vi "refresh table model.vi"(7 "engine configuration":refnum<class "engine configuration.lvclass">, 8 "error in":errorcluster, 9 "avail tags":refnum<vi>, 10 "chan table":refnum<vi>, 11 "bin datalogger configuration":refnum<class "Binary datalogger configuration.lvclass">) -> (0 "error out":errorcluster, 3 "bin datalogger configuration out":refnum<class "Binary datalogger configuration.lvclass">, 5 "engine configuration out":refnum<class "engine configuration.lvclass">)   [LabVIEW 2013, in "Binary datalogger editor node.lvclass"]
uses:
  Binary datalogger editor node.lvclass
  module/configuration/Binary datalogger configuration.lvclass
  <vilib>/NI/Module Execution Interface/Engine Configuration/engine configuration.lvclass
  <vilib>/NI/Configuration Framework/serializable configuration/NISE_CEF_serializable configuration.lvclass/NISE_CEF_serializable configuration.ctl
  module/configuration/Binary datalogger configuration.lvclass/Binary datalogger configuration.ctl
  <vilib>/NI/Tag Bus/tag/tag descriptor.lvclass/tag descriptor.ctl
  <vilib>/NI/Module Execution Interface/Engine Configuration/engine configuration.lvclass/engine configuration.ctl
  <vilib>/NI/Tag Bus/tag/write tag name.vi
  <vilib>/NI/Tag Bus/tag/read tag name.vi
  <vilib>/NI/Tag Bus/tag/read data type.vi
  <vilib>/NI/Configuration Framework/serializable configuration/Read UID.vi
  module/configuration/Read channels.vi
  <vilib>/Utility/LVClass/Get LV Class Name.vi
  <vilib>/NI/Configuration Framework/error generator/NISE_error generator.vi
  <vilib>/NI/Tag Bus Module Framework/channel/TBM channel.lvclass
  <vilib>/NI/Tag Bus/tag/tag descriptor.lvclass
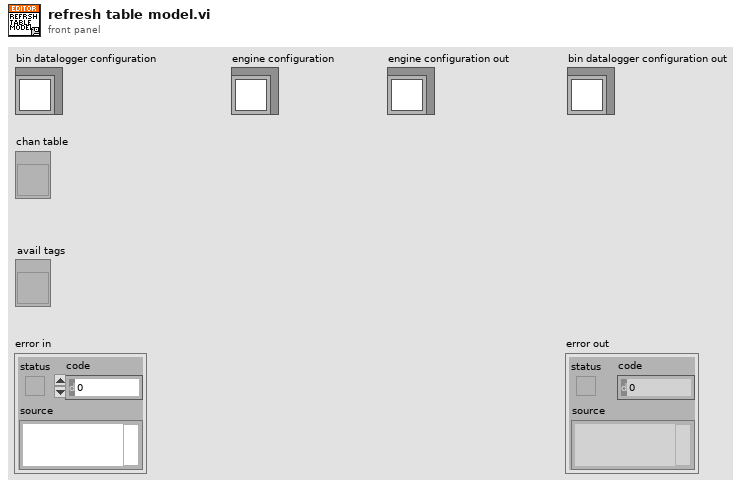
[diagram p1: front panel]
types:
  T1 = typedef "tag bus.lvlib/tag descriptor.lvclass/Data Type.ctl" = enum16{"Double", "Single", "I64", "I32", "I16", "I8", "U64", "U32", "U16", "U8", "Boolean", "String", "Array of Double", "Array of Single", "Array of I64", "Array of I32", "Array of I16", "Array of I8", "Array of U64", "Array of U32", "Array of U16", "Array of U8", "Array of Boolean", "Array of String"}
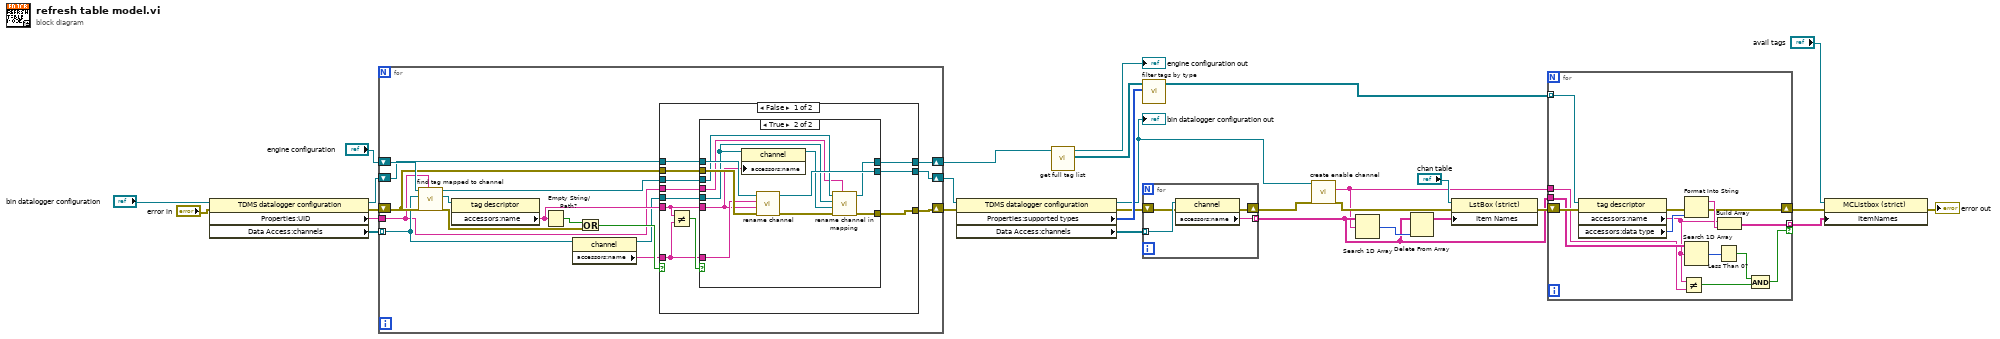
[diagram p0: block diagram]
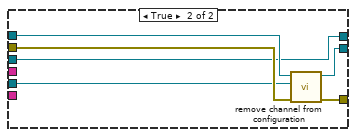
[diagram p3: hidden frame]
diagram:
  n1 = property class="TDMS datalogger configuration"(reference="bin datalogger configuration", error in="error in") -> (reference out=w24:refnum<class "Binary datalogger configuration.lvclass">, error out=w26:errorcluster, "Properties:UID"=w20:string, "Data Access:channels"=w27:refnum<class "TBM channel.lvclass">[])
  n2 = for {
    tunnel: w27 -> [w37] mode=indexing
    shift-right: [w32] -> w8
    shift-left: "engine configuration" -> [w45]
    shift-right: [w42] -> w23
    shift-left: w24 -> [w40]
    tunnel: w20 -> [w31]
    shift-right: [w41] -> w22
    shift-left: w26 -> [w38]
    n3 = call <vilib>:"find tag mapped to channel.vi"("owner"=w31, "error in"=w38, "channel"=w37, "engine configuration in"=w45) -> ("error out"=w36:errorcluster, "tag"=w44:refnum<class "tag descriptor.lvclass">, "engine configuration out"=w33:refnum<class "engine configuration.lvclass">)  [unwired: 5 in]
    n4 = property class="tag descriptor"(reference=w44) -> ("accessors:name"=w34:string)  [unwired: 1 in, 2 out]
    n5 = Empty String/Path?(string/path=w34) -> (empty?=w43:bool)
    n6 = property class="channel"(reference=w37) -> (reference out=w30:refnum<class "TBM channel.lvclass">, "accessors:name"=w35:string)  [unwired: 1 in, 1 out]
    n7 = Or(x=w43, y=w36) -> (x .or. y?=w39:bool)
    n8 = case shown="False" w39 {
      tunnel: [w53 w77] -> w42
      tunnel: [w56 w76] -> w41
      tunnel: w38 -> [w55 w75]
      tunnel: w40 -> [w54 w74]
      tunnel: w30 -> [w46 w73]
      tunnel: w35 -> [w51 _]
      tunnel: w34 -> [w50 _]
      tunnel: w33 -> [w49 w72]
      tunnel: [w48 w72] -> w32
      tunnel: w31 -> [w47 _]
      frame False {
        n9 = Not Equal?(x=w50, y=w51) -> (x != y?=w52:bool)
        n10 = case shown="True" w52 {
          tunnel: [w59 w64] -> w56
          tunnel: w55 -> [w59 w70]
          tunnel: w54 -> [w58 w71]
          tunnel: [w58 w69] -> w53
          tunnel: w51 -> [_ w68]
          tunnel: w50 -> [_ w61]
          tunnel: w49 -> [w57 w67]
          tunnel: [w57 w66] -> w48
          tunnel: w47 -> [_ w63]
          tunnel: w46 -> [_ w62]
          frame False {
          }
          frame True {
            n11 = property class="channel"(reference=w62, "accessors:name"=w61) -> (reference out=w60:refnum<class "TBM channel.lvclass">)  [unwired: 1 in, 1 out]
            n12 = call "rename channel.vi"("error in"=w70, "new name"=w61, "old name"=w68, "bin datalogger configuration in"=w71) -> ("error out"=w65:errorcluster, "bin datalogger configuration out"=w69:refnum<class "Binary datalogger configuration.lvclass">)  [unwired: 6 in]
            n13 = call <vilib>:"rename channel in mapping.vi"("owner ID"=w63, "error in"=w65, "new channel"=w60, "old channel"=w62, "engine configuration in"=w67) -> ("error out"=w64:errorcluster, "engine configuration out"=w66:refnum<class "engine configuration.lvclass">)  [unwired: 5 in]
          }
        }
      }
      frame True {
        n14 = call "remove channel from configuration.vi"("error in"=w75, "TBM channel in"=w73, "bin datalogger configuration in"=w74) -> ("error out"=w76:errorcluster, "bin datalogger configuration out"=w77:refnum<class "Binary datalogger configuration.lvclass">)  [unwired: 7 in]
      }
    }
  }
  n15 = property class="TDMS datalogger configuration"(reference=w23, error in=w22) -> (reference out=w1:refnum<class "Binary datalogger configuration.lvclass">, error out=w18:errorcluster, "Properties:supported types"=w21:T1[], "Data Access:channels"=w19:refnum<class "TBM channel.lvclass">[])
  "bin datalogger configuration out" <- w1
  n16 = call <vilib>:"get full tag list.vi"("engine configuration in"=w8) -> ("tag list"=w6:refnum<class "tag descriptor.lvclass">[], "engine configuration out"=→"engine configuration out":refnum<class "engine configuration.lvclass">)  [unwired: 9 in]
  n17 = call <vilib>:"filter tags by type.vi"("allowable types"=w21, "tags in"=w6) -> ("filtered tags"=w15:refnum<class "tag descriptor.lvclass">[])  [unwired: 9 in]
  n18 = for {
    tunnel: w19 -> [w81] mode=indexing
    shift-right: [w80] -> w4
    shift-left: w18 -> [w79]
    tunnel: [w78] -> w5 mode=indexing
    n19 = property class="channel"(reference=w81, error in=w79) -> (error out=w80:errorcluster, "accessors:name"=w78:string)  [unwired: 1 out]
  }
  n20 = call "create enable channel.vi"("error in"=w4, "bin datalogger configuration"=w1) -> ("error out"=w3:errorcluster, "enable channel name"=w2:string)  [unwired: 7 in, 1 out]
  n21 = Search 1D Array(1D array=w5, element=w2) -> (index of element=w17:i32)  [unwired: 1 in]
  n22 = Delete From Array(array=w5, index=w17) -> (array with subset deleted=w16:string[])  [unwired: 1 in, 1 out]
  n23 = property class="LstBox (strict)"(reference="chan table", error in=w3, "Item Names"=w16) -> (error out=w14:errorcluster)  [unwired: 1 out]
  n24 = for {
    tunnel: w15 -> [w93] mode=indexing
    shift-right: [w90] -> w13
    shift-left: w14 -> [w92]
    tunnel: [w89] -> w12 mode=indexing if=w85
    tunnel: w5 -> [w88]
    tunnel: w2 -> [w83]
    n25 = property class="tag descriptor"(reference=w93, error in=w92) -> (error out=w91:errorcluster, "accessors:name"=w84:string, "accessors:data type"=w94:T1)  [unwired: 1 out]
    n26 = Not Equal?(x=w84, y=w83) -> (x != y?=w82:bool)
    n27 = Format Into String(error in=w91, w94) -> (resulting string=w95:string, error out=w90:errorcluster)  [unwired: 2 in]
    n28 = Search 1D Array(1D array=w88, element=w84) -> (index of element=w87:i32)  [unwired: 1 in]
    n29 = Less Than 0?(x=w87) -> (x < 0?=w86:bool)
    n30 = Build Array(w84, w95) -> (w89:string[])
    n31 = Compound Arithmetic op=AND(w86, w82) -> (w85:bool)
  }
  n32 = property class="MCListbox (strict)"(reference="avail tags", error in=w13, "ItemNames"=w12) -> (error out=→"error out":errorcluster)  [unwired: 1 out]
